vi "Initialize & Card test.vi"(8 "error in (no error)":errorcluster, 11 "ShotsPerPoint":u16=100) -> (0 "error out":errorcluster, 3 "TenAccumulate":cluster{"MassX":dbl[], "TenScans":sgl[]}(graph))   [LabVIEW 2013]
uses:
  libtiepie.dll
panel:
  in  "StopCard":bool
  in  "Takedata":bool
  in  "MassTime":bool
  out "MassX":dbl[](array[numeric])
  in  "a2":dbl=1.8e-05
  in  "a1":dbl=0.0064
  in  "a0":dbl=-0.25
  out "TimeX":dbl[](array[numeric])
  out "PresentShot":i32
  out "Intensity_Total":sgl[](array[numeric])
  out "Intensity_SinglePoint":sgl[](array[numeric])
  out "getdata":u64
  out "InitializeCardErr":errorcluster
  out "Channel 1":bool
  in  "Channel 1_Range":dbl(ring)=4.0 items=["80 V"=80.0, "40 V"=40.0, "20 V"=20.0, "8 V"=8.0, "4 V"=4.0, "2 V"=2.0, "800 mV"=0.8, "400 mV"=0.4, "200 mV"=0.2]
  in  "CH1_Coupling":u64(ring)=1 items=["Volt DC"=1, "Volt AC"=2, "Ampere DC"=4, "Ampere AC"=8, "Ohm"=16]
  in  "Record Length/Samples":u64=50000
  in  "Sample Frequency/Hz":i32=200000000
  out "channelCount":u16
  out "TpDeviceHandle_t":u32
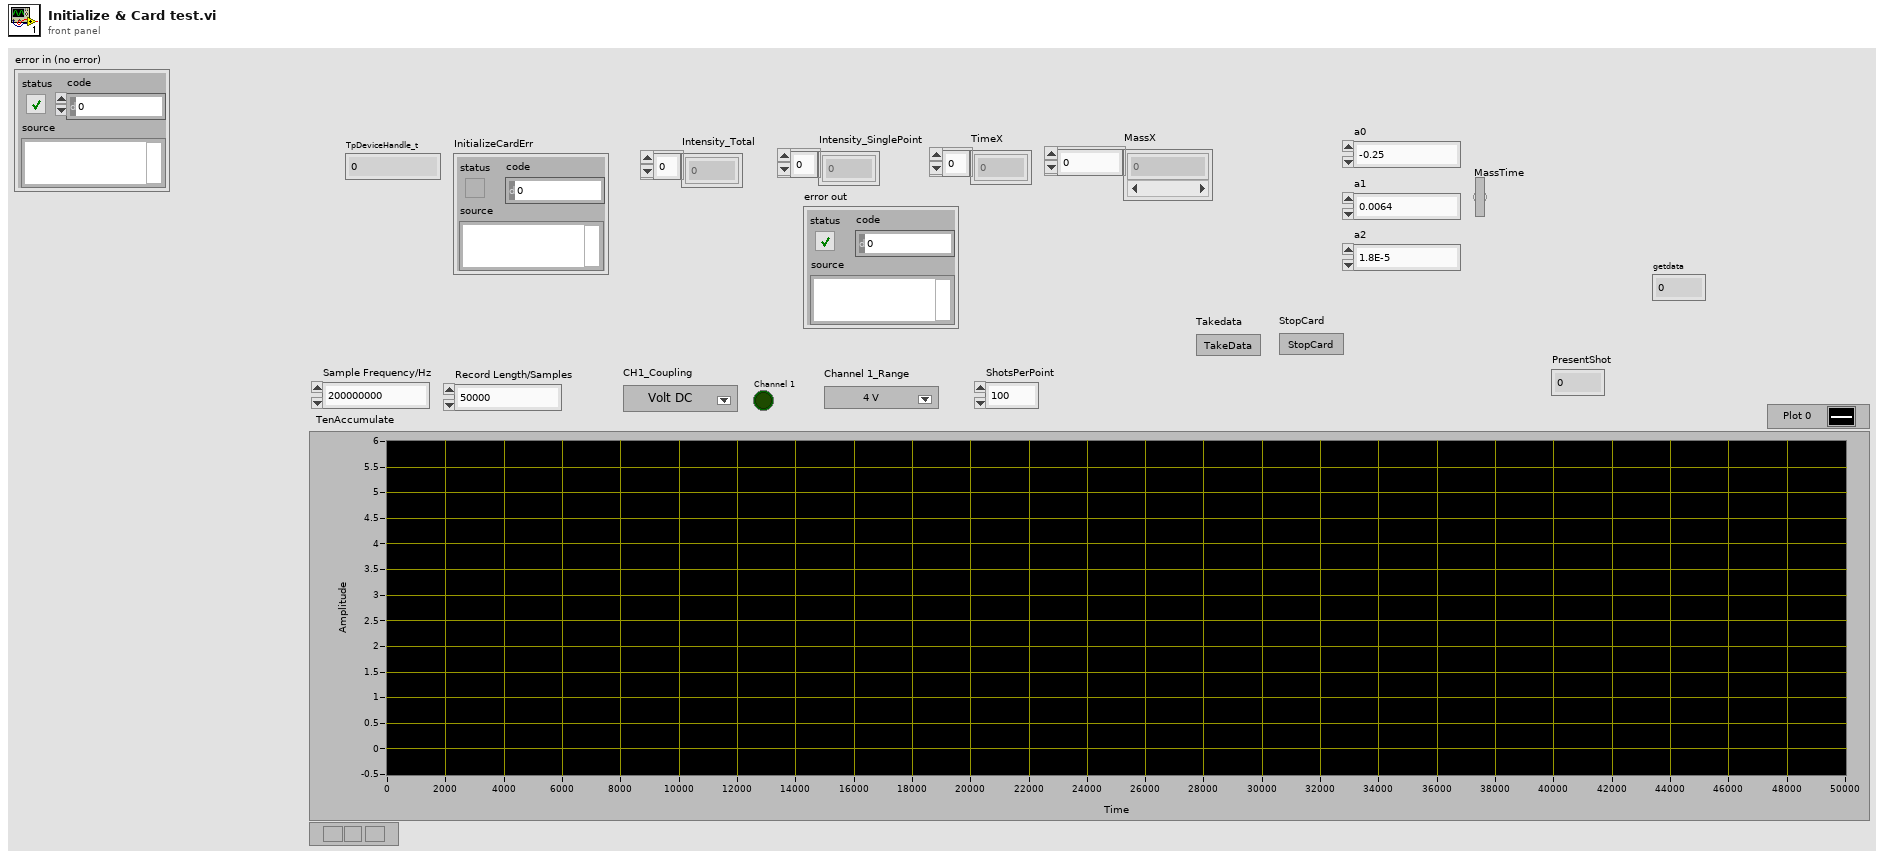
[diagram p1: front panel]
types:
  T1 = cluster{"MassX":dbl[], "Intensity_SinglePoint":sgl[]}
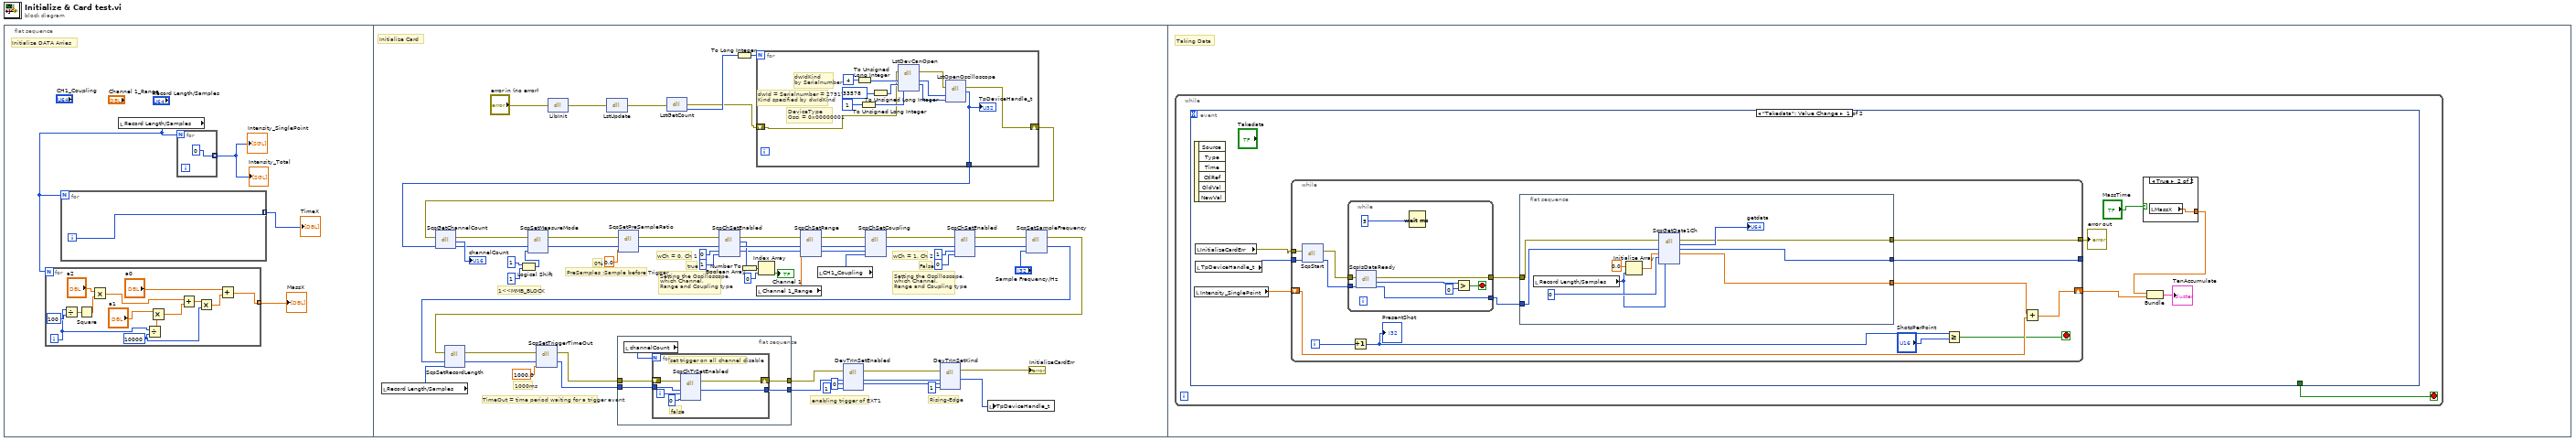
[diagram p0: block diagram]
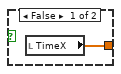
[diagram p2: hidden frame]
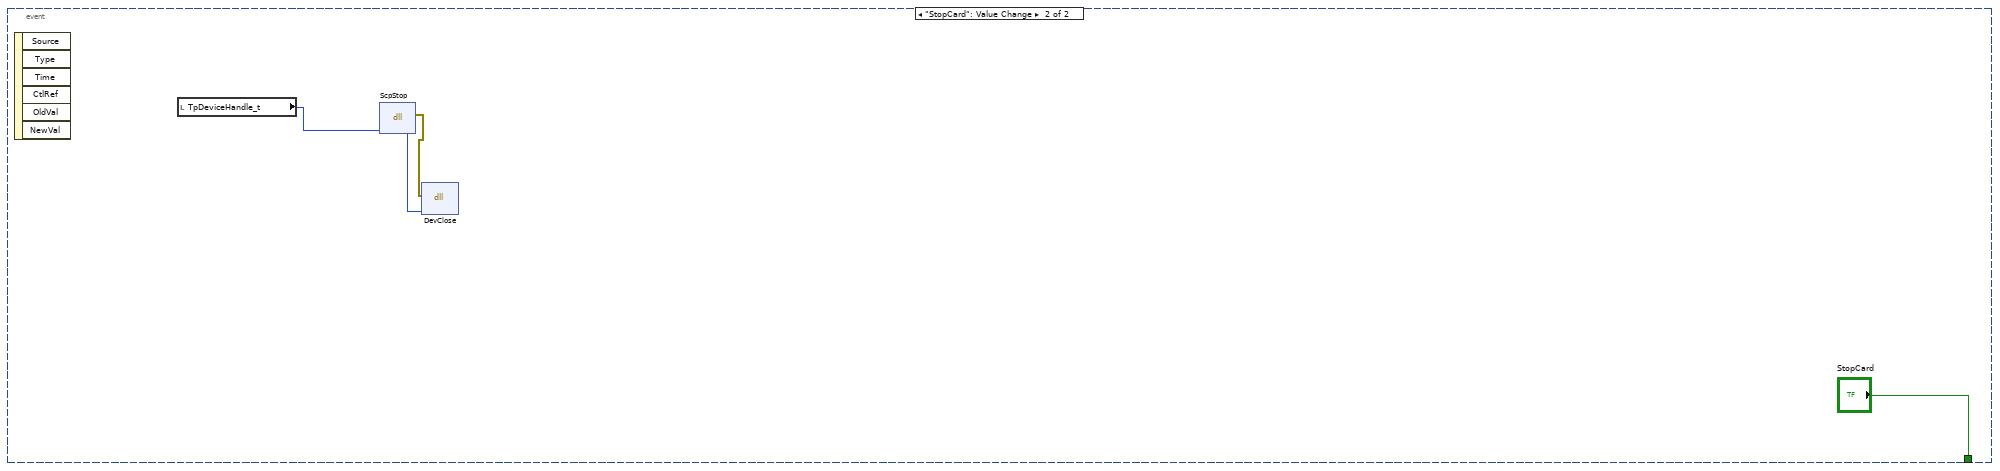
[diagram p3: hidden frame]
diagram:
  n1 = flat-sequence {
    frame #0 {
      # "Initialize DATA Arries"
      n2 = local read "Record Length/Samples"() -> (w4:u64)
      n3 = for {
        N: w4 -> [_]
        tunnel: [w8] -> w2 mode=indexing
        i -> [w12]
        w6 = 10000
        n4 = Divide(x=w12, y=100) -> (x/y=w15:dbl)
        n5 = Square(x=w15) -> (x^2=w17:dbl)
        n6 = Multiply(x="a2", y=w17) -> (x*y=w11:dbl)
        n7 = Divide(x=w12, y=w6) -> (x/y=w13:dbl)
        n8 = Multiply(x="a1", y=w13) -> (x*y=w10:dbl)
        n9 = Add(x=w11, y=w10) -> (x+y=w7:dbl)
        n10 = Multiply(x=w7, y=w6) -> (x*y=w5:dbl)
        n11 = Add(x="a0", y=w5) -> (x+y=w8:dbl)
      }
      "MassX" <- w2
      n12 = for {
        N: w4 -> [_]
        tunnel: [w19] -> w3 mode=indexing
        i -> [w19]
      }
      "TimeX" <- w3
      n13 = for {
        N: w4 -> [_]
        tunnel: [0] -> w1 mode=indexing
      }
      "Intensity_SinglePoint" <- w1
      "Intensity_Total" <- w1
    }
    frame #1 {
      # "Rising-Edge"
      # "enabling trigger of EXT1"
      # "1000ms"
      # "TimeOut = time period waiting for a trigger event"
      # "Setting the Oscilloscope,\nwhich Channel, \nRange and Coupling type"
      # "wCh = 1. Ch 2"
      # "False"
      # "Setting the Oscilloscope,\nwhich Channel, \nRange and Coupling type"
      # "wCh = 0, Ch 1"
      # "true"
      # "0%"
      # "PreSamples :Sample before Trigger"
      # "1<<MMB_BLOCK"
      # "Initialize Card"
      n14 = local read "Record Length/Samples"() -> (w22:u64)
      n15 = Logical Shift(y=u32 1, x=u32 1 ("y")) -> (x << y=w50:u32)
      n16 = dll-call lib="PTH1Fabs CUsers82158DesktopTOF software\t数据卡\nlibtiepie.dll" fn="LibInit"(error in="error in (no error)") -> (error out=w77:errorcluster)  [unwired: 3 in, 1 out]
      n17 = dll-call lib="PTH1Fabs CUsers82158DesktopTOF software\t数据卡\nlibtiepie.dll" fn="LstUpdate"(error in=w77) -> (error out=w27:errorcluster)  [unwired: 3 in, 1 out]
      n18 = flat-sequence {
        tunnel: w34 -> [w83]
        tunnel: w35 -> [w82]
        tunnel: [w80] -> w43
        tunnel: [w79] -> w44
        frame #0 {
          n19 = local read "channelCount"() -> (w81:u16)
          n20 = for {
            N: w81 -> [_]
            tunnel: w83 -> [w86]
            shift-right: [w85] -> w80
            shift-left: w82 -> [w87]
            tunnel: [w84] -> w79
            i -> [w89]
            # "set trigger on all channel disable"
            # "false"
            n21 = dll-call lib="PTH1Fabs CUsers82158DesktopTOF software\t数据卡\nlibtiepie.dll" fn="ScpChTrSetEnabled"(error in=w87, "TpDeviceHandle_t"=w86, "wCh"=w89, "bEnable"=u8 0) -> (error out=w85:errorcluster, "TpDeviceHandle_t"=w84:u32)  [unwired: 5 in, 1 out]
          }
        }
      }
      n22 = dll-call lib="PTH1Fabs CUsers82158DesktopTOF software\t数据卡\nlibtiepie.dll" fn="LstGetCount"(error in=w27) -> (error out=w28:errorcluster, "Count"=w29:u32)  [unwired: 2 in, 1 out]
      n23 = To Long Integer(number=w29) -> (32bit integer=w78:i32)
      n24 = for {
        N: w78 -> [_]
        shift-right: [w92] -> w33
        shift-left: w28 -> [w91]
        tunnel: [w90] -> w32
        # "DeviceType\nOsci = 0x00000001"
        # "dwId = Serialnumber = 27917\nKind specified by dwIdKind"
        # "dwIdKind\nby Serialnumber"
        n25 = To Unsigned Long Integer(number=4) -> (unsigned 32bit integer=w100:u32)
        n26 = To Unsigned Long Integer(number=1) -> (unsigned 32bit integer=w98:u32)
        n27 = To Unsigned Long Integer(number=33578) -> (unsigned 32bit integer=w96:u32)
        n28 = dll-call lib="PTH1Fabs CUsers82158DesktopTOF software\t数据卡\nlibtiepie.dll" fn="LstDevCanOpen"(error in=w91, "dwIdKind"=w100, "dwId"=w96, "dwDeviceType"=w98) -> (error out=w93:errorcluster, "dwIdKind"=w94:u32, "dwId"=w95:u32)  [unwired: 4 in, 1 out]
        n29 = dll-call lib="PTH1Fabs CUsers82158DesktopTOF software\t数据卡\nlibtiepie.dll" fn="LstOpenOscilloscope"(error in=w93, "dwIdKind"=w94, "dwId"=w95) -> (error out=w92:errorcluster, "TpDeviceHandle_t"=w90:u32)  [unwired: 4 in, 1 out]
        "TpDeviceHandle_t" <- w90
      }
      n30 = dll-call lib="PTH1Fabs CUsers82158DesktopTOF software\t数据卡\nlibtiepie.dll" fn="ScpGetChannelCount"(error in=w33, "TpDeviceHandle_t"=w32) -> (error out=w46:errorcluster, "channelCount"=→"channelCount":u16, "TpDeviceHandle_t"=w45:u32)  [unwired: 2 in, 1 out]
      n31 = dll-call lib="PTH1Fabs CUsers82158DesktopTOF software\t数据卡\nlibtiepie.dll" fn="ScpSetMeasureMode"(error in=w46, "TpDeviceHandle_t"=w45, "dwMeasureMode"=w50) -> (error out=w56:errorcluster, "TpDeviceHandle_t"=w57:u32)  [unwired: 4 in, 1 out]
      n32 = dll-call lib="PTH1Fabs CUsers82158DesktopTOF software\t数据卡\nlibtiepie.dll" fn="ScpSetPreSampleRatio"(error in=w56, "TpDeviceHandle_t"=w57, "dPreSampleRatio"=0.0) -> (error out=w52:errorcluster, "TpDeviceHandle_t"=w54:u32)  [unwired: 4 in, 1 out]
      n33 = dll-call lib="PTH1Fabs CUsers82158DesktopTOF software\t数据卡\nlibtiepie.dll" fn="ScpChSetEnabled"(error in=w52, "TpDeviceHandle_t"=w54, "wCh"=u16 0, "bEnable"=u8 1) -> (error out=w61:errorcluster, "Enabled"=w69:u8, "TpDeviceHandle_t"=w70:u32, "wCh"=w62:u16)  [unwired: 3 in, 1 out]
      n34 = Number To Boolean Array(number=w69) -> (Boolean array=w66:bool[])
      n35 = local read "Channel 1_Range"() -> (w65:dbl)
      n36 = Index Array(array=w66, index=0) -> (element=→"Channel 1":bool)
      n37 = dll-call lib="PTH1Fabs CUsers82158DesktopTOF software\t数据卡\nlibtiepie.dll" fn="ScpChSetRange"(error in=w61, "TpDeviceHandle_t"=w70, "wCh"=w62, "dRange"=w65) -> (error out=w71:errorcluster, "TpDeviceHandle_t"=w73:u32, "wCh"=w72:u16)  [unwired: 4 in, 1 out]
      n38 = local read "CH1_Coupling"() -> (w64:u64)
      n39 = dll-call lib="PTH1Fabs CUsers82158DesktopTOF software\t数据卡\nlibtiepie.dll" fn="DevTrInSetEnabled"(error in=w43, "hDevice"=w44, "wInput"=u16 0, "enable"=u8 1) -> (error out=w40:errorcluster, "hDevice"=w39:u32, "wInput"=w38:u16)  [unwired: 4 in, 1 out]
      n40 = dll-call lib="PTH1Fabs CUsers82158DesktopTOF software\t数据卡\nlibtiepie.dll" fn="ScpChSetCoupling"(error in=w71, "TpDeviceHandle_t"=w73, "wCh"=w72, "qwCoupling"=w64) -> (error out=w53:errorcluster, "TpDeviceHandle_t"=w76:u32)  [unwired: 5 in, 1 out]
      n41 = dll-call lib="PTH1Fabs CUsers82158DesktopTOF software\t数据卡\nlibtiepie.dll" fn="DevTrInSetKind"(error in=w40, "hDevice"=w39, "wInput"=w38, "qwkind"=u64 1) -> (error out=→"InitializeCardErr":errorcluster, "hDevice"=w30:u32)  [unwired: 5 in, 1 out]
      n42 = dll-call lib="PTH1Fabs CUsers82158DesktopTOF software\t数据卡\nlibtiepie.dll" fn="ScpChSetEnabled"(error in=w53, "TpDeviceHandle_t"=w76, "wCh"=u16 1, "bEnable"=u8 0) -> (error out=w58:errorcluster, "TpDeviceHandle_t"=w59:u32)  [unwired: 5 in, 1 out]
      n43 = local write "TpDeviceHandle_t"(w30) -> ()
      n44 = dll-call lib="PTH1Fabs CUsers82158DesktopTOF software\t数据卡\nlibtiepie.dll" fn="ScpSetSampleFrequency"(error in=w58, "TpDeviceHandle_t"=w59, "SampleFrequency"="Sample Frequency/Hz") -> (error out=w24:errorcluster, "TpDeviceHandle_t"=w23:u32)  [unwired: 4 in, 1 out]
      n45 = dll-call lib="PTH1Fabs CUsers82158DesktopTOF software\t数据卡\nlibtiepie.dll" fn="ScpSetRecordLength"(error in=w24, "TpDeviceHandle_t"=w23, "qwRecordLength"=w22) -> (error out=w26:errorcluster, "TpDeviceHandle_t"=w25:u32)  [unwired: 4 in, 1 out]
      n46 = dll-call lib="PTH1Fabs CUsers82158DesktopTOF software\t数据卡\nlibtiepie.dll" fn="ScpSetTriggerTimeOut"(error in=w26, "TpDeviceHandle_t"=w25, "dTimeOut"=1000.0) -> (error out=w35:errorcluster, "TpDeviceHandle_t"=w34:u32)  [unwired: 4 in, 1 out]
    }
    frame #2 {
      # "Taking Data"
      n47 = while {
        stop <- w102 stop-if-true
        n48 = event shown="[0] \"Takedata\": Value Change" {
          selector: _ -> [_ _]
          dyn-events: _ -> [_ _]
          timeout: _ -> [_ _]
          tunnel: [_ "StopCard"] -> w102
          event "Takedata": Value Change {
            n49 = event-data() -> ()  [unwired: 1 in, 6 out]
            n50 = local read "Intensity_SinglePoint"() -> (w110:sgl[])
            n51 = local read "InitializeCardErr"() -> (w106:errorcluster)
            n52 = local read "TpDeviceHandle_t"() -> (w105:u32)
            n53 = while {
              tunnel: w106 -> [w127]
              tunnel: w105 -> [w126]
              tunnel: [w125] -> w103
              tunnel: [w124] -> _
              shift-right: [w119] -> w104
              shift-left: w110 -> [w120]
              i -> [w118]
              stop <- w117 stop-if-true
              n54 = dll-call lib="PTH1Fabs CUsers82158DesktopTOF software\t数据卡\nlibtiepie.dll" fn="ScpStart"(error in=w127, "TpDeviceHandle_t"=w126) -> (error out=w123:errorcluster, "TpDeviceHandle_t"=w122:u32)  [unwired: 3 in, 1 out]
              n55 = while {
                tunnel: w123 -> [w135]
                tunnel: w122 -> [w134]
                tunnel: [w133] -> w114
                tunnel: [w132] -> w113
                stop <- w129 stop-if-true
                n56 = dll-call lib="PTH1Fabs CUsers82158DesktopTOF software\t数据卡\nlibtiepie.dll" fn="ScpIsDataReady"(error in=w135, "TpDeviceHandle_t"=w134) -> (error out=w133:errorcluster, "DataReady"=w130:u8, "TpDeviceHandle_t"=w132:u32)  [unwired: 2 in, 1 out]
                n57 = Wait (ms)(milliseconds to wait=u32 5) -> ()  [unwired: 1 out]
                n58 = Greater?(x=w130, y=0 ("index")) -> (0:w129:bool)
              }
              n59 = Increment(x=w118) -> (x+1=w116:i32)
              "PresentShot" <- w116
              n60 = flat-sequence {
                tunnel: [w142] -> w125
                tunnel: [w141] -> w124
                tunnel: [w140] -> w121
                tunnel: w114 -> [w137]
                tunnel: w113 -> [w136]
                frame #0 {
                  n61 = local read "Record Length/Samples"() -> (w138:u64)
                  n62 = Initialize Array(0.0 ("element"), w138) -> (w145:dbl[])
                  n63 = dll-call lib="PTH1Fabs CUsers82158DesktopTOF software\t数据卡\nlibtiepie.dll" fn="ScpGetData1Ch"(error in=w137, "TpDeviceHandle_t"=w136, "pBufferCh1"=w145, "qwStartIndex"=u64 0, "qwSampleCount"=w138) -> (error out=w142:errorcluster, "return type"=→"getdata":u64, "TpDeviceHandle_t"=w141:u32, "pBufferCh1"=w140:sgl[])  [unwired: 4 in, 1 out]
                }
              }
              n64 = Greater Or Equal?(x=w116, y="ShotsPerPoint") -> (x >= y?=w117:bool)
              n65 = Add(x=w121, y=w120) -> (x+y=w119:sgl[])
            }
            "error out" <- w103
            n66 = case shown="True" "MassTime" {
              tunnel: [w111 w112] -> w107
              frame False {
                n67 = local read "TimeX"() -> (w111:dbl[])
              }
              frame True {
                n68 = local read "MassX"() -> (w112:dbl[])
              }
            }
            n69 = Bundle("MassX"=w107, "Intensity_SinglePoint"=w104) -> (→"TenAccumulate":T1)  [unwired: 1 in]
          }
          event "StopCard": Value Change {
            n70 = event-data() -> ()  [unwired: 1 in, 6 out]
            n71 = local read "TpDeviceHandle_t"() -> (w146:u32)
            n72 = dll-call lib="PTH1Fabs CUsers82158DesktopTOF software\t数据卡\nlibtiepie.dll" fn="ScpStop"("TpDeviceHandle_t"=w146) -> (error out=w148:errorcluster, "TpDeviceHandle_t"=w147:u32)  [unwired: 4 in, 1 out]
            n73 = dll-call lib="PTH1Fabs CUsers82158DesktopTOF software\t数据卡\nlibtiepie.dll" fn="DevClose"(error in=w148, "hDevice"=w147) -> ()  [unwired: 4 in, 2 out]
          }
        }
      }
    }
  }
